vi "复位定时器.vi"(8 "error in (no error)":errorcluster caption="错误输入（无错误）", 11 "定时器类 输入":refnum<class "定时器类.lvclass">) -> (0 "error out":errorcluster caption="错误输出", 3 "定时器类 输出":refnum<class "定时器类.lvclass">)   [LabVIEW 2014, in "定时器类.lvclass"]
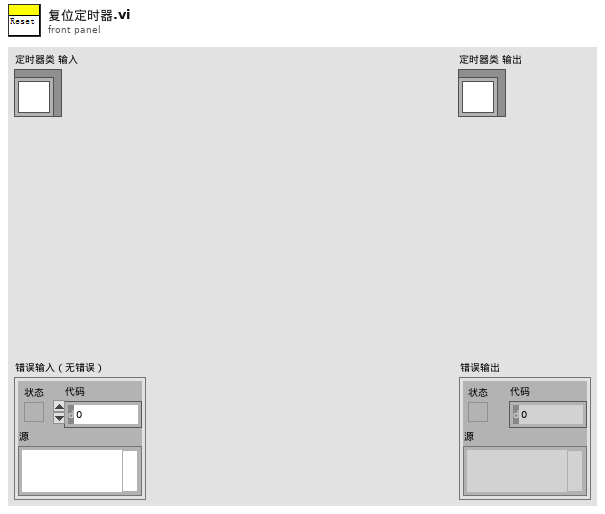
[diagram p1: front panel]
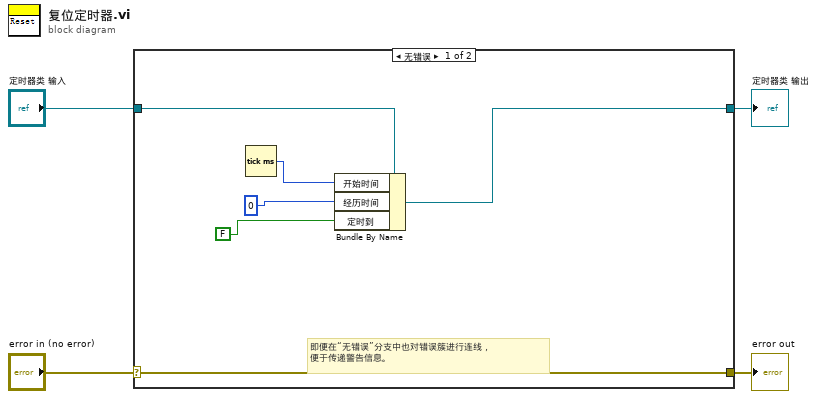
[diagram p0: block diagram]
diagram:
  n1 = case shown="无错误" "error in (no error)" {
    selector: "error in (no error)" -> [w10 w12]
    tunnel: [w10 w12] -> w3
    tunnel: [w5 w11] -> w1
    tunnel: "定时器类 输入" -> [w6 w11]
    frame No Error {
      # "即便在“无错误”分支中也对错误簇进行连线，\n便于传递警告信息。"
      n2 = Tick Count (ms)() -> (millisecond timer value=w7:u32)
      n3 = Bundle By Name(cluster=w6, "开始时间"=w7, "经历时间"=0, "定时到"=FALSE) -> (w5:refnum<class "定时器类.lvclass">)
    }
    frame Error {
    }
  }
  "error out" <- w3
  "定时器类 输出" <- w1
